vi "Initialize Settings 1.0.vi"(8 "error in (no error)":errorcluster, 11 "settings 1.0":cluster{"key":string, "value":string}[](array[cluster])) -> (0 "error out":errorcluster, 3 "configuration 1.0":cluster{"processor":i32, "priority offset":i16}={"processor"=-2, "priority offset"=0})   [LabVIEW 2017, in "DSF Core.lvlib" / "Thread Configuration.lvclass"]
uses:
  Thread Configuration.lvclass
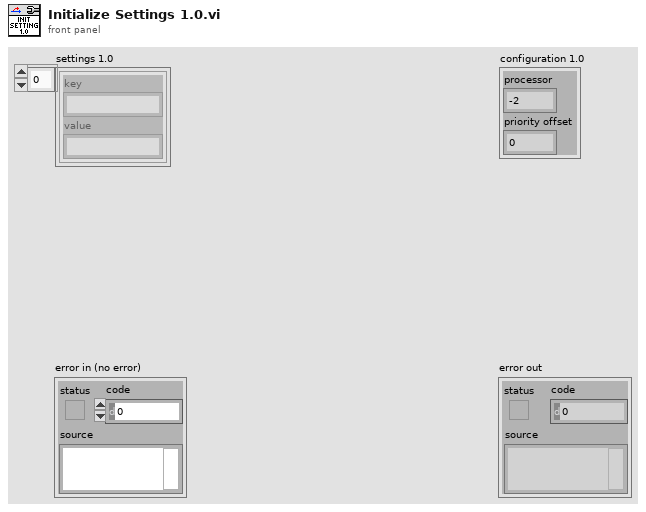
[diagram p1: front panel]
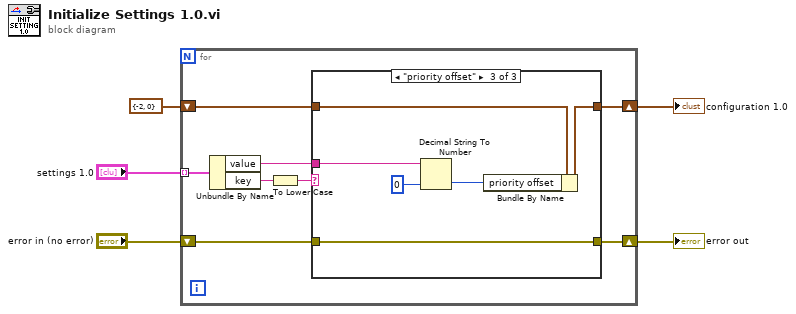
[diagram p0: block diagram]
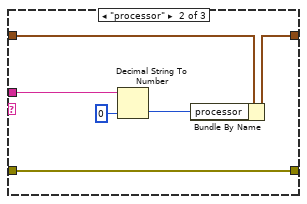
[diagram p3: hidden frame]
diagram:
  n1 = for {
    shift-right: [w8] -> w5
    shift-left: cluster{"processor":i32, "priority offset":i16} {"processor"=-2, "priority offset"=0} ("configuration 1.0") -> [w9]
    tunnel: "settings 1.0" -> [w13] mode=indexing
    shift-right: [w6] -> w4
    shift-left: "error in (no error)" -> [w7]
    n2 = Unbundle By Name(w13) -> ("value"=w10:string, "key"=w12:string)
    n3 = To Lower Case(string=w12) -> (all lower case string=w11:string)
    n4 = case shown="\"priority offset\"" w11 {
      tunnel: w10 -> [_ w17 w23]
      tunnel: w9 -> [w15 w21 w27]
      tunnel: [w15 w20 w26] -> w8
      tunnel: w7 -> [w14 w19 w25]
      tunnel: [w14 w19 w25] -> w6
      frame Default {
        # "Unknown setting."
      }
      frame "processor" {
        n5 = Decimal String To Number(string=w17, default (0L)=0 ("default (0 I32)")) -> (number=w18:i32)  [unwired: 1 in, 1 out]
        n6 = Bundle By Name(cluster=w21, "processor"=w18) -> (w20:cluster{"processor":i32, "priority offset":i16})
      }
      frame "priority offset" {
        n7 = Decimal String To Number(string=w23, default (0L)=i16 0 ("default (0 I32)")) -> (number=w24:i16)  [unwired: 1 in, 1 out]
        n8 = Bundle By Name(cluster=w27, "priority offset"=w24) -> (w26:cluster{"processor":i32, "priority offset":i16})
      }
    }
  }
  "error out" <- w4
  "configuration 1.0" <- w5
